vi "MGI VI Tree.vi"(11 "MGI Error Reporter Base.lvclass":refnum<class "MGI Error Reporter Base.lvclass">) -> ()   [LabVIEW 2020, in "MGI Error Reporter Base.lvclass"]
doc: "This VI documents the MGI Error Reporter Base Class.\nSee Block Diagram for documentation.\n\nAuthored by Shawn Walpole\nsupport@mooregoodideas.com\nwww.mooregoodideas.com\n\nCopyright (c) 2013, Moore Good Ideas, Inc.\n\nAll rights reserved.\n\nRedistribution and use in source and binary forms, with or without modification, are permitted provided that the following conditions are met:\n\n * Redistributions of source code must retain the above copyright notice, this list of conditions and the following disclaimer.\n * Redistributions in binary form must reproduce the above copyright notice, this list of conditions and the following disclaimer in the documentation and/or other materials provided with the distribution.\n * Neither the name of Moore Good Ideas, Inc. nor the names of its contributors may be used to endorse or promote products derived from this software without specific prior written permission.\n\nTHIS SOFTWARE IS PROVIDED BY THE COPYRIGHT HOLDERS AND CONTRIBUTORS \"AS IS\" AND ANY EXPRESS OR IMPLIED WARRANTIES, INCLUDING, BUT NOT LIMITED TO, THE IMPLIED WARRANTIES OF MERCHANTABILITY AND FITNESS FOR A PARTICULAR PURPOSE ARE DISCLAIMED. IN NO EVENT SHALL THE COPYRIGHT OWNER OR CONTRIBUTORS BE LIABLE FOR ANY DIRECT, INDIRECT, INCIDENTAL, SPECIAL, EXEMPLARY, OR CONSEQUENTIAL DAMAGES (INCLUDING, BUT NOT LIMITED TO, PROCUREMENT OF SUBSTITUTE GOODS OR SERVICES; LOSS OF USE, DATA, OR PROFITS; OR BUSINESS INTERRUPTION) HOWEVER CAUSED AND ON ANY THEORY OF LIABILITY, WHETHER IN CONTRACT, STRICT LIABILITY, OR TORT (INCLUDING NEGLIGENCE OR OTHERWISE) ARISING IN ANY WAY OUT OF THE USE OF THIS SOFTWARE, EVEN IF ADVISED OF THE POSSIBILITY OF SUCH DAMAGE."
uses:
  <userlib>/_MGI/Error Reporter/MGI Error Reporter Base/MGI Error Reporter Base.lvclass
  <userlib>/_MGI/Error Reporter/MGI Error Reporter Base/Protected/MGI Cmd Enum.ctl
panel:
  # "See Block Diagram for Class Documentation"
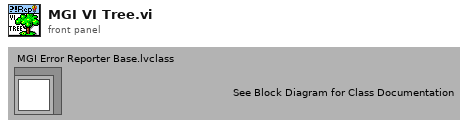
[diagram p1: front panel]
types:
  T1 = typedef "MGI Error Reporter Base.lvclass/MGI Cmd Enum.ctl" = enum16{"Quit", "Show UI"}
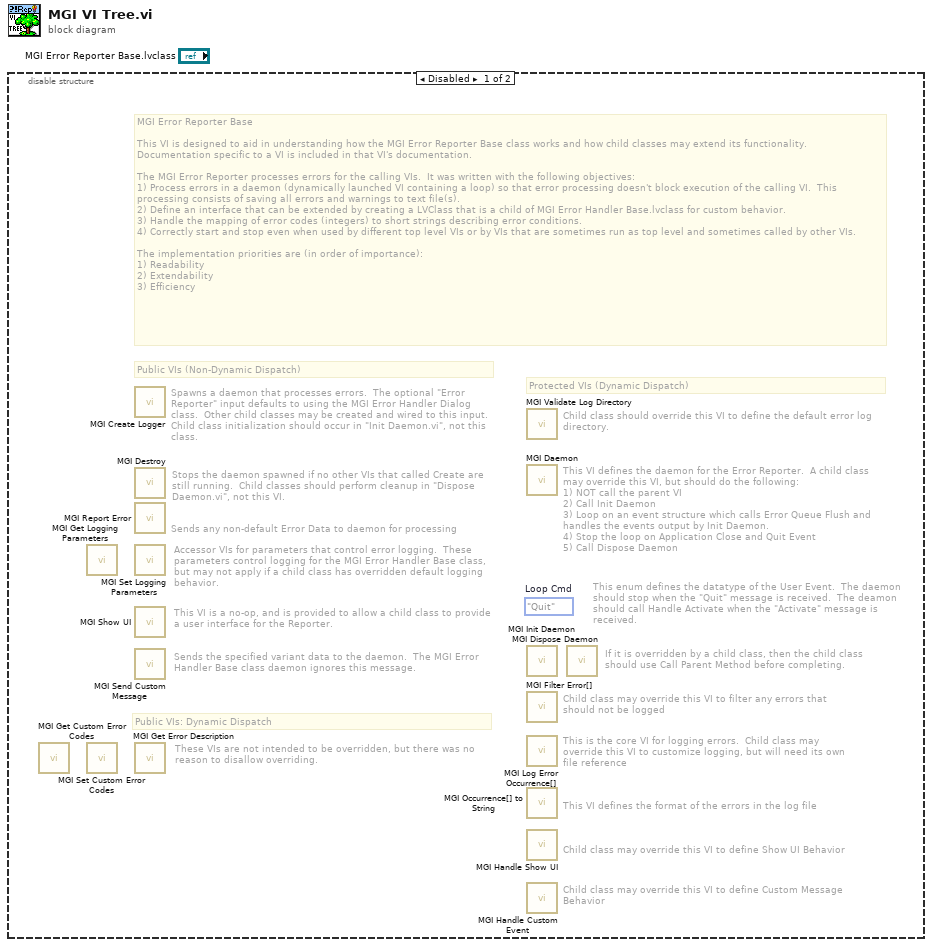
[diagram p0: block diagram]
diagram:
  n1 = disable-structure shown="Disabled" {
    frame Disabled {
      (unwired) MGI_Cmd_Enum."Quit"  # Loop Cmd
      # "Child class may override this VI to define Custom Message Behavior"
      # "Child class may override this VI to define Show UI Behavior"
      # "This VI defines the format of the errors in the log file"
      # "This is the core VI for logging errors.  Child class may override this VI to customize logging, but will need its own file reference"
      # "Child class may override this VI to filter any errors that should not be logged"
      # "Child class should override this VI to define the default error log directory."
      # "If it is overridden by a child class, then the child class should use Call Parent Method before completing."
      # "This enum defines the datatype of the User Event.  The daemon should stop when the \"Quit\" message is received.  The deamon should call Handle Activate when the \"Activate\" message is received."
      # "This VI defines the daemon for the Error Reporter.  A child class may override this VI, but should do the following:\n1) NOT call the parent VI\n2) Call Init Daemon\n3) Loop on an event structure which calls Error Queue Flush and handles the events output by Init Daemon.\n4) Stop the loop on Application Close and Quit Event\n5) Call Dispose Daemon"
      # "MGI Error Reporter Base\n\nThis VI is designed to aid in understanding how the MGI Error Reporter Base class works and how child classes may extend its functionality.  Documentation specific to a VI is included in that VI's documentation.\n\nThe MGI Error Reporter processes errors for the calling VIs.  It was written with the following objectives:\n1) Process errors in a daemon (dynamically launched VI containing a loop) so that error processing doesn't block execution of the calling VI.  This processing consists of saving all errors and warnings to text file(s).\n2) Define an interface that can be extended by creating a LVClass that is a child of MGI Error Handler Base.lvclass for custom behavior.\n3) Handle the mapping of error codes (integers) to short strings describing error conditions.\n4) Correctly start and stop even when used by different top level VIs or by VIs that are sometimes run as top level and sometimes called by other VIs.\n\nThe implementation priorities are (in order of importance):\n1) Readability\n2) Extendability\n3) Efficiency"
      # "These VIs are not intended to be overridden, but there was no reason to disallow overriding."
      # "Sends the specified variant data to the daemon.  The MGI Error Handler Base class daemon ignores this message."
      # "This VI is a no-op, and is provided to allow a child class to provide a user interface for the Reporter."
      # "Accessor VIs for parameters that control error logging.  These parameters control logging for the MGI Error Handler Base class, but may not apply if a child class has overridden default logging behavior."
      # "Sends any non-default Error Data to daemon for processing"
      # "Stops the daemon spawned if no other VIs that called Create are still running.  Child classes should perform cleanup in \"Dispose Daemon.vi\", not this VI."
      # "Spawns a daemon that processes errors.  The optional \"Error Reporter\" input defaults to using the MGI Error Handler Dialog class.  Other child classes may be created and wired to this input.  Child class initialization should occur in \"Init Daemon.vi\", not this class."
      # "Public VIs: Dynamic Dispatch"
      # "Protected VIs (Dynamic Dispatch)"
      # "Public VIs (Non-Dynamic Dispatch)"
      n2 = call-dynamic "MGI Get Custom Error Codes.vi"() -> ()  [unwired: 10 in, 2 out]
      n3 = call <userlib>:"MGI Get Logging Parameters.vi"() -> ()  [unwired: 9 in, 3 out]
      n4 = call-dynamic "MGI Set Custom Error Codes.vi"() -> ()  [unwired: 11 in, 1 out]
      n5 = call <userlib>:"MGI Create Logger.vi"() -> ()  [unwired: 9 in, 3 out]
      n6 = call <userlib>:"MGI Destroy.vi"() -> ()  [unwired: 11 in, 1 out]
      n7 = call <userlib>:"MGI Report Error.vi"() -> ()  [unwired: 11 in, 1 out]
      n8 = call <userlib>:"MGI Set Logging Parameters.vi"() -> ()  [unwired: 11 in, 1 out]
      n9 = call <userlib>:"MGI Show UI.vi"() -> ()  [unwired: 11 in, 1 out]
      n10 = call <userlib>:"MGI Send Custom Message.vi"() -> ()  [unwired: 11 in, 1 out]
      n11 = call <userlib>:"MGI Get Error Description.vi"() -> ()  [unwired: 10 in, 2 out]
      n12 = call-dynamic "MGI Validate Log Directory.vi"() -> ()  [unwired: 10 in, 2 out]
      n13 = call-dynamic "MGI Daemon.vi"() -> ()  [unwired: 11 in, 1 out]
      n14 = call-dynamic "MGI Init Daemon.vi"() -> ()  [unwired: 9 in, 3 out]
      n15 = call-dynamic "MGI Filter Error[].vi"() -> ()  [unwired: 10 in, 2 out]
      n16 = call-dynamic "MGI Log Error Occurrence[].vi"() -> ()  [unwired: 10 in, 2 out]
      n17 = call-dynamic "MGI Occurrence[] to String.vi"() -> ()  [unwired: 9 in, 3 out]
      n18 = call-dynamic "MGI Handle Show UI.vi"() -> ()  [unwired: 10 in, 2 out]
      n19 = call-dynamic "MGI Handle Custom Event.vi"() -> ()  [unwired: 10 in, 2 out]
      n20 = call-dynamic "MGI Dispose Daemon.vi"() -> ()  [unwired: 11 in, 1 out]
    }
    frame Enabled {
    }
  }
